vi "DT_Pre.vi"(9 "rotation angle":dbl, 10 "Y":dbl[](array[numeric]), 11 "X":dbl[](array[numeric])) -> (1 "scale factor":dbl, 2 "Rev Index":i32[](array[numeric]), 3 "Points":cluster{"x":dbl, "y":dbl, "index":i32}[](array[cluster]))   [LabVIEW 2017, in "NI_AAL_Geometry.lvlib"]
uses:
  <vilib>/Analysis/NI_AAL_Geometry.lvlib
  <vilib>/Analysis/coordinate.llb/2D Cartesian Coordinate Rotation (Array).vi
  <vilib>/Analysis/NI_AALPro.lvlib
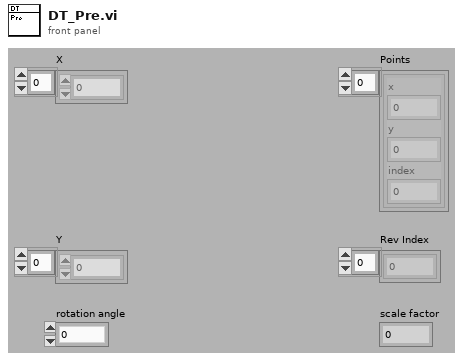
[diagram p1: front panel]
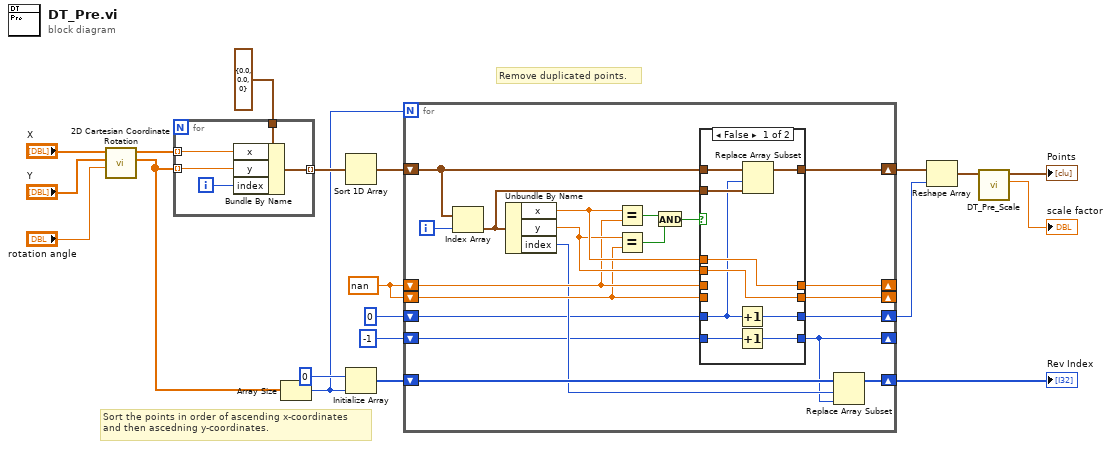
[diagram p0: block diagram]
diagram:
  w17 = nan
  # "Remove duplicated points."
  # "Sort the points in order of ascending x-coordinates\nand then ascedning y-coordinates."
  n1 = call-poly <vilib>:"2D Cartesian Coordinate Rotation.vi"("theta"="rotation angle", "Y"="Y", "X"="X") -> ("Y Out"=w2:dbl[], "X Out"=w4:dbl[])  [unwired: 6 in, 1 out]
  n2 = for {
    tunnel: w4 -> [w24] mode=indexing
    tunnel: w2 -> [w23] mode=indexing
    tunnel: cluster{"x":dbl, "y":dbl, "index":i32} {"x"=0.0, "y"=0.0, "index"=0} ("point") -> [w25]
    tunnel: [w21] -> w19 mode=indexing
    i -> [w22]
    n3 = Bundle By Name(cluster=w25, "x"=w24, "y"=w23, "index"=w22) -> (w21:cluster{"x":dbl, "y":dbl, "index":i32})
  }
  n4 = Array Size(array=w2) -> (size(s)=w9:i32)
  n5 = Sort 1D Array(array=w19) -> (sorted array=w18:cluster{"x":dbl, "y":dbl, "index":i32}[])
  n6 = Initialize Array(0 ("element"), w9) -> (w13:i32[])
  n7 = for {
    N: w9 -> [_]
    shift-right: [w35] -> w16
    shift-left: w18 -> [w28]
    shift-right: [w38] -> _
    shift-left: w17 -> [w40]
    shift-right: [w37] -> _
    shift-left: w17 -> [w39]
    shift-right: [w36] -> w15
    shift-left: 0 -> [w31]
    shift-right: [w33] -> w12
    shift-left: w13 -> [w34]
    shift-right: [w29] -> _
    shift-left: -1 -> [w30]
    i -> [w27]
    n8 = Index Array(array=w28, index=w27) -> (element=w26:cluster{"x":dbl, "y":dbl, "index":i32})
    n9 = Unbundle By Name(w26) -> ("x"=w42:dbl, "y"=w41:dbl, "index"=w32:i32)
    n10 = Equal?(x=w42, y=w40) -> (x = y?=w45:bool)
    n11 = Equal?(x=w41, y=w39) -> (x = y?=w44:bool)
    n12 = And(x=w45, y=w44) -> (x .and. y?=w43:bool)
    n13 = case shown="False" w43 {
      tunnel: w28 -> [w52 w57]
      tunnel: w31 -> [w50 w56]
      tunnel: w42 -> [w54 _]
      tunnel: w41 -> [w53 _]
      tunnel: w40 -> [_ w59]
      tunnel: w39 -> [_ w58]
      tunnel: [w54 w59] -> w38
      tunnel: [w53 w58] -> w37
      tunnel: w26 -> [w51 _]
      tunnel: [w49 w56] -> w36
      tunnel: [w48 w57] -> w35
      tunnel: w30 -> [w47 w55]
      tunnel: [w46 w55] -> w29
      frame False {
        n14 = Increment(x=w50) -> (x+1=w49:i32)
        n15 = Increment(x=w47) -> (x+1=w46:i32)
        n16 = Replace Array Subset(array=w52, new element=w51, index=w50) -> (w48:cluster{"x":dbl, "y":dbl, "index":i32}[])
      }
      frame True {
      }
    }
    n17 = Replace Array Subset(array=w34, new element=w29, index=w32) -> (w33:i32[])
  }
  "Rev Index" <- w12
  n18 = Reshape Array(w16, w15) -> (w8:cluster{"x":dbl, "y":dbl, "index":i32}[])
  n19 = call <vilib>:"DT_Pre_Scale.vi"("Points In"=w8) -> ("scale factor"=→"scale factor":dbl, "Points Out"=→"Points":cluster{"x":dbl, "y":dbl, "index":i32}[])  [unwired: 9 in]
